vi "Teleop Tester.vi"() -> ()   [LabVIEW 2020]
uses:
  <vilib>/Analysis/coordinate.llb/2D Cartesian Coordinate Rotation (Scalar).vi
  <vilib>/Analysis/NI_AALPro.lvlib
panel:
  out "?":picture
  out "RR":bool=TRUE
  # "Teleop Tester:\n\n1.) Plug In Joystick\n2.) Swap out Teleop Emulator VI in\nthe block diagram\n3.) Drive!\n3.) If you lose the robot, click on the\npicture and the robot will move there"
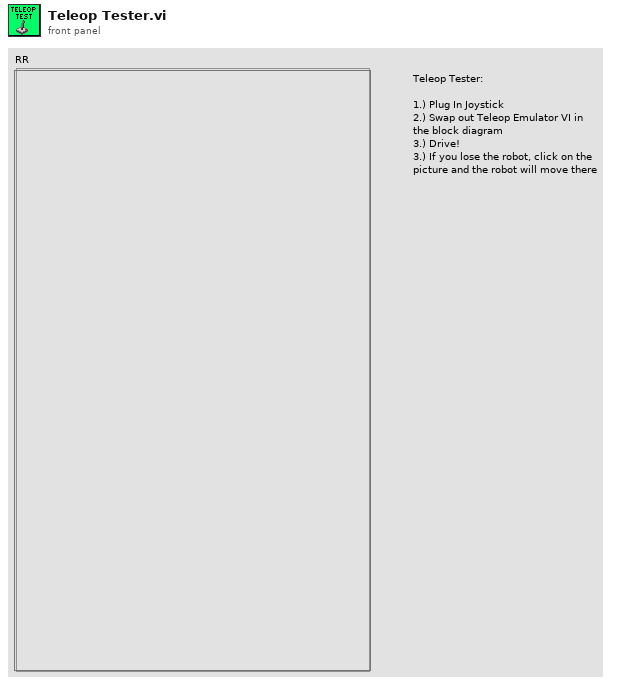
[diagram p1: front panel]
types:
  T1 = typedef "LVPositionTypeDef.ctl" = cluster{"Left":i32, "Top":i32}
  T2 = typedef "LVBoundsTypeDef.ctl" = cluster{"Width":u32, "Height":u32}
  T3 = typedef "Robot Velocities.ctl" = cluster{"vx":dbl, "vy":dbl, "w":dbl}
  T4 = typedef "LVPoint32TypeDef.ctl" = cluster{"Horizontal":i32, "Vertical":i32}
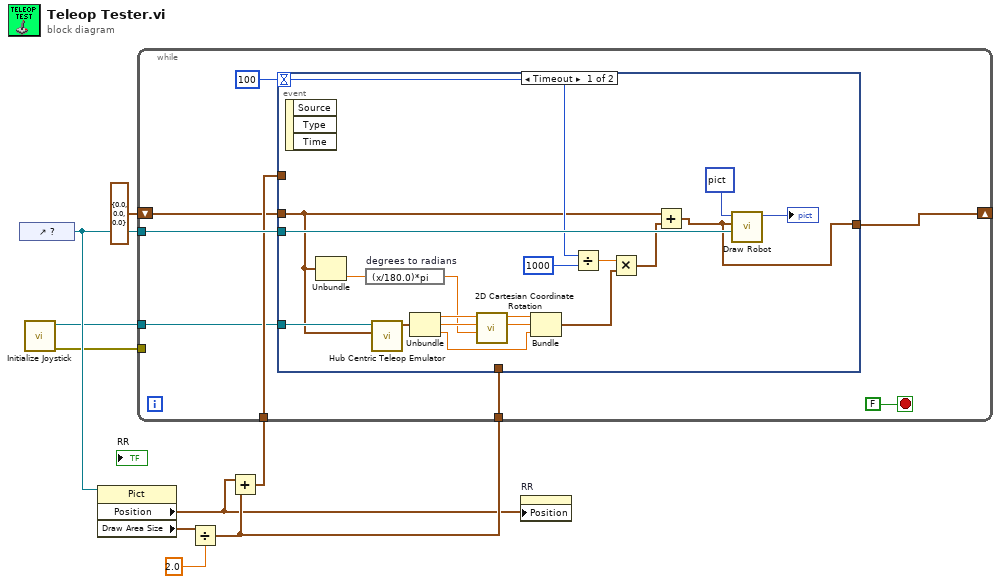
[diagram p0: block diagram]
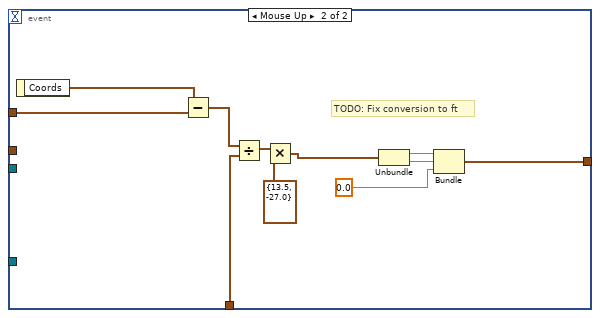
[diagram p2: hidden frame]
diagram:
  n1 = control-ref of="?"() -> (w9:refnum<vi>)
  n2 = call <vilib>:"Initialize Joystick.vi"() -> ("error out"=w1:errorcluster, "device ID"=w2:refnum<k1>)  [unwired: 10 in]
  n3 = property class="Pict"(reference=w9) -> ("Position"=w4:T1, "Draw Area Size"=w8:T2)  [unwired: 1 in, 2 out]
  n4 = Divide(x=w8, y=2.0) -> (x/y=w5:cluster{"Width":dbl, "Height":dbl})
  n5 = Add(x=w4, y=w5) -> (x+y=w6:cluster{dbl, dbl})
  n6 = while {
    tunnel: w9 -> [w15]
    tunnel: w6 -> [w14]
    tunnel: w5 -> [w13]
    shift-right: [w12] -> _
    shift-left: cluster{dbl, dbl, dbl} {0.0, 0.0, 0.0} -> [w11]
    tunnel: w2 -> [w10]
    tunnel: w1 -> [_]
    stop <- FALSE stop-if-true
    n7 = event shown="[0] Timeout" {
      selector: _ -> [_ _]
      dyn-events: _ -> [_ _]
      timeout: 100 -> [w31 _]
      tunnel: w15 -> [w34 _]
      tunnel: w14 -> [_ w47]
      tunnel: w13 -> [_ w41]
      tunnel: [w33 w37] -> w12
      tunnel: w11 -> [w18 _]
      tunnel: w10 -> [w19 _]
      event Timeout {
        n8 = event-data() -> ()  [unwired: 1 in, 3 out]
        n9 = Unbundle(w18) -> (w21:dbl)  [unwired: 2 out]
        n10 = expression code="(x/180.0)*pi" "degrees to radians"(w21) -> (w22:dbl)
        n11 = call "Hub Centric Teleop Emulator.vi"("Current Pose"=w18, "device ID"=w19) -> ("Robot Velocities"=w20:T3)  [unwired: 9 in]
        n12 = Unbundle(w20) -> ("vx"=w28:dbl, "vy"=w27:dbl, "w"=w24:dbl)
        n13 = call-poly <vilib>:"2D Cartesian Coordinate Rotation.vi"("theta"=w22, "y"=w27, "x"=w28) -> ("y out"=w25:dbl, "x out"=w26:dbl)  [unwired: 6 in, 1 out]
        n14 = Bundle("x out"=w26, "y out"=w25, "w"=w24) -> (w23:cluster{"x out":dbl, "y out":dbl, "w":dbl})  [unwired: 1 in]
        n15 = Divide(x=w31, y=1000) -> (x/y=w29:dbl)
        n16 = Multiply(x=w29, y=w23) -> (x*y=w32:cluster{"x out":dbl, "y out":dbl, "w":dbl})
        n17 = Add(x=w18, y=w32) -> (x+y=w33:cluster{dbl, dbl, dbl})
        n18 = call "Draw Robot.vi"("Picture  Reference"=w34, "Pose"=w33, "Picture In"=picture data[5B]) -> ("Picture Out"=→"?":picture)  [unwired: 8 in]
      }
      event Mouse Up {
        # "TODO: Fix conversion to ft"
        n19 = event-data() -> ("Coords"=w46:T4)  [unwired: 1 in]
        n20 = Subtract(x=w46, y=w47) -> (x-y=w42:cluster{dbl, dbl})
        n21 = Divide(x=w42, y=w41) -> (x/y=w40:cluster{dbl, dbl})
        n22 = Multiply(x=w40, y=cluster{dbl, dbl} {13.5, -27.0}) -> (x*y=w38:cluster{dbl, dbl})
        n23 = Unbundle(w38) -> (w45:dbl, w44:dbl)
        n24 = Bundle(w45, w44, 0.0) -> (w37:cluster{dbl, dbl, dbl})  [unwired: 1 in]
      }
    }
  }
  n25 = property on="RR" class="Bool (strict)"("Position"=w4) -> ()  [unwired: 2 in, 2 out]
